vi "GetProperties.vi"(8 "error in":errorcluster, 11 "VisaResourceName in":refnum<class "VisaResourceName.lvclass">) -> (0 "error out":errorcluster, 3 "VisaResourceName out":refnum<class "VisaResourceName.lvclass">)   [LabVIEW 2014, in "VisaResourceName.lvclass"]
uses:
  VisaResourceName.lvclass
  VisaResourceName.lvclass/VisaResourceName.ctl
  IOName/IOName.lvclass
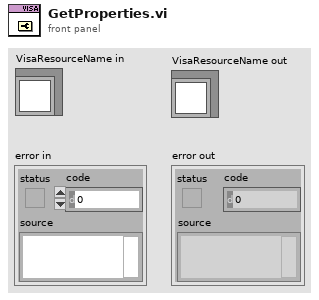
[diagram p1: front panel]
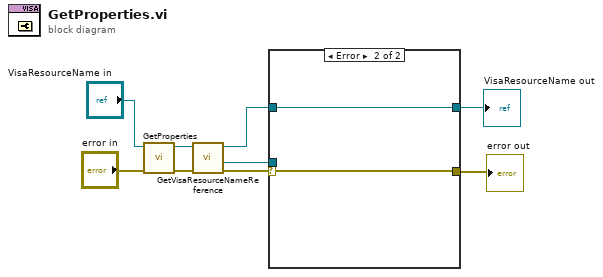
[diagram p0: block diagram]
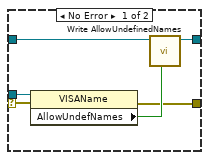
[diagram p2: hidden frame]
diagram:
  n1 = call-parent "GetProperties.vi"("error in"="error in", "IOName in"="VisaResourceName in") -> ("error out"=w6:errorcluster, "IOName out"=w7:refnum<class "VisaResourceName.lvclass">)  [unwired: 8 in]
  n2 = call "GetVisaResourceNameReference.vi"("error in"=w6, "VisaResourceName in"=w7) -> ("error out"=w5:errorcluster, "Visa Resource reference"=w4:refnum<vi>, "VisaResourceName out"=w3:refnum<class "VisaResourceName.lvclass">)  [unwired: 7 in]
  n3 = case shown="Error" w5 {
    selector: w5 -> [w14 w17]
    tunnel: w4 -> [w15 _]
    tunnel: w3 -> [w13 w16]
    tunnel: [w11 w17] -> w1
    tunnel: [w10 w16] -> w2
    frame No Error {
      n4 = property class="VISAName"(reference=w15, error in=w14) -> (error out=w11:errorcluster, "AllowUndefNames"=w12:bool)  [unwired: 1 out]
      n5 = call "Write AllowUndefinedNames.vi"("Allow Undefined Names"=w12, "VisaResourceName in"=w13) -> ("VisaResourceName out"=w10:refnum<class "VisaResourceName.lvclass">)  [unwired: 7 in]
    }
    frame Error {
    }
  }
  "error out" <- w1
  "VisaResourceName out" <- w2
